vi "UI_Loading_Unit_Test2.vi"() -> ()   [LabVIEW 2014]
panel:
  in  "修改":bool
  in  "加载单元液位过低":bool caption="液位过低"
  in  "加载单元液位过高":bool caption="液位过高"
  in  "加载单元回油过滤器堵塞":bool caption="回油过滤器堵塞"
  in  "加载单元供油过滤器堵塞":bool caption="供油过滤器堵塞"
  out "轴向液压缸加载压力":u16
  out "径向液压缸加载压力":u16
  in  "退出":bool
  in  "系统启动":bool
  out "轴向液压缸加载压力'":dbl(graph) caption="轴向液压缸加载压力"
  out "径向液压缸加载压力'":dbl(graph) caption="径向液压缸加载压力"
  in  "轴向载荷F2":u16
  in  "径向载荷F1":u16
  out "加载单元调试状态":bool
  # "加载单元独立调试"
  # "监测参数"
  # "报警信息"
  # "传\n感\n器"
  # "单\n元\n系\n统"
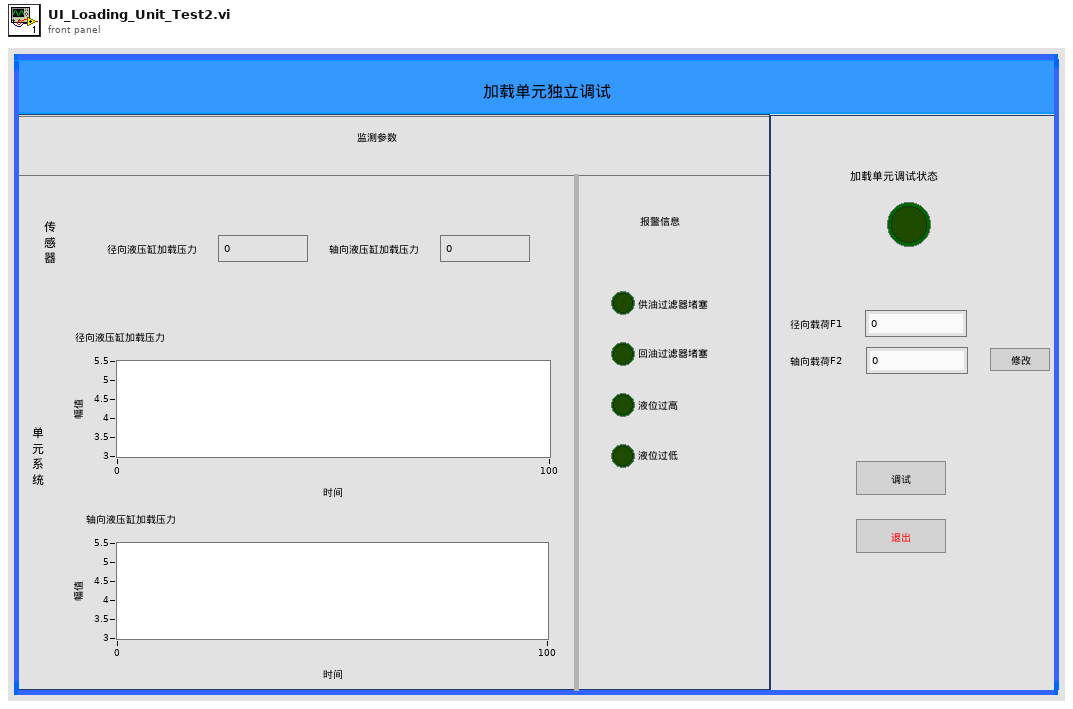
[diagram p1: front panel]
types:
  T1 = cluster{"径向油缸加载压力":u16, "轴向油缸加载压力":u16, "油箱1油液温度":u16, "润滑油温度":u16, "油箱2油液温度":u16, "试验轴承供油压力":u16, "试验轴承供油流量":u16, "陪试轴承供油流量":u16, "陪试轴承供油压力":u16, "陪试轴承供油温度":u16, "液压子系统状态字":cluster{"加载单元":cluster{"供油过滤器堵塞报警":bool, "回油过滤器堵塞报警":bool, "液位过高报警":bool, "液位过低报警":bool}, "试验轴承单元":cluster{"加热装置异常报警":bool, "油箱1液位过高报警":bool, "油箱1液位过低报警":bool, "油箱2液位过高报警":bool, "油箱2液位过低报警":bool, "供油过滤器堵塞报警":bool, "循环回路过滤器堵塞报警":bool, "回油过滤器堵塞报警":bool}, "陪试轴承单元":cluster{"供油过滤器1堵塞报警":bool, "供油过滤器2堵塞报警":bool, "回油过滤器堵塞报警":bool, "油箱液位过高报警":bool, "油箱液位过低报警":bool}}}
  T2 = cluster{"供油过滤器堵塞报警":bool, "回油过滤器堵塞报警":bool, "液位过高报警":bool, "液位过低报警":bool}
  T3 = cluster{"时间":timestamp, "陪试轴承润滑单元出油温度1":sgl[], "陪试轴承润滑单元出油温度2":sgl[], "轴承外圈温度":sgl[], "出油温度":sgl[], "摩擦力1":sgl[], "摩擦力2":sgl[], "径向油缸力":sgl[], "轴向油缸力":sgl[], "转速":sgl[]}
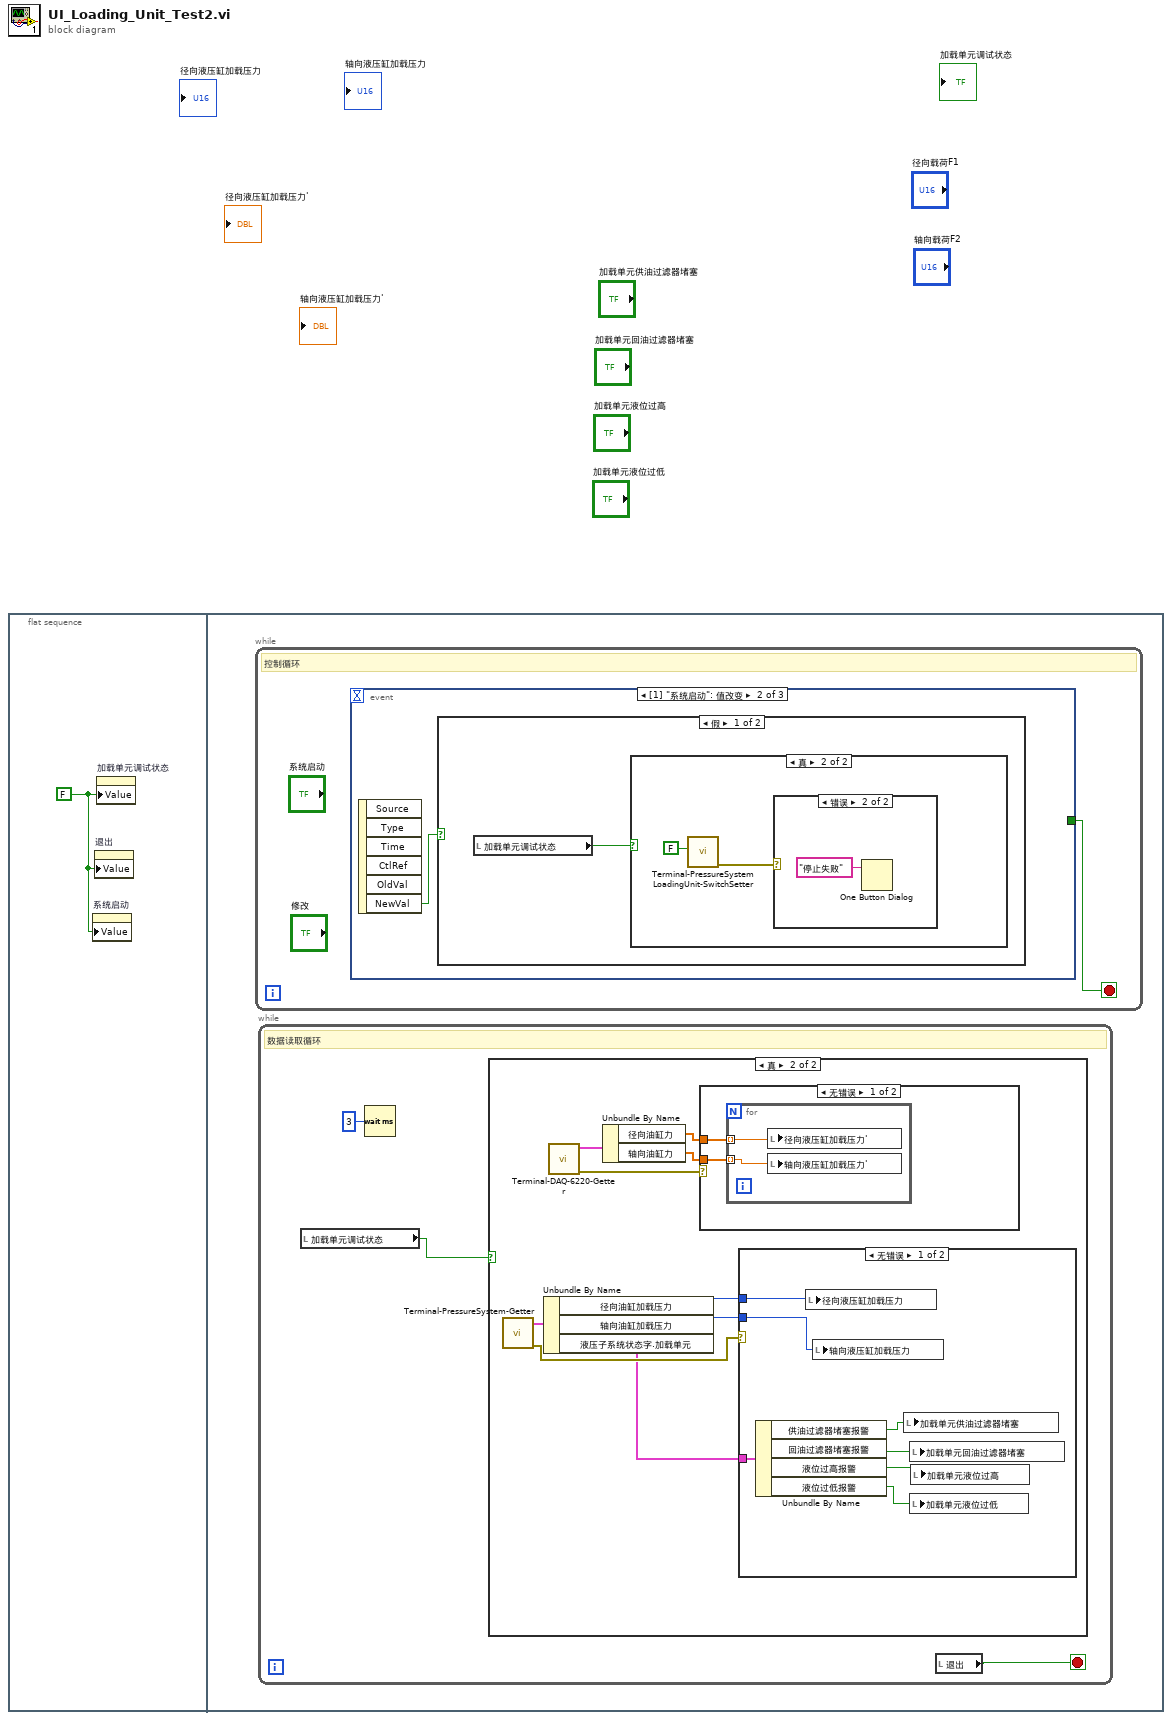
[diagram p0: block diagram]
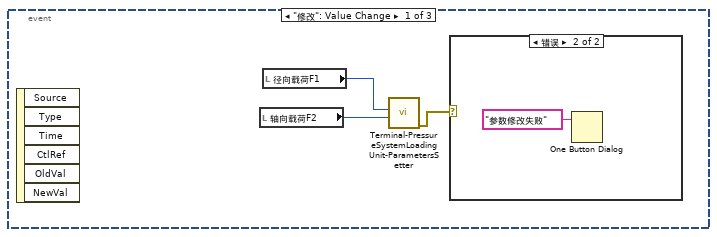
[diagram p5: hidden frame]
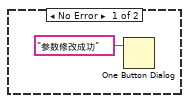
[diagram p6: hidden frame]
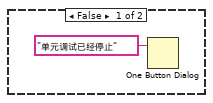
[diagram p7: hidden frame]
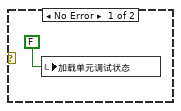
[diagram p8: hidden frame]
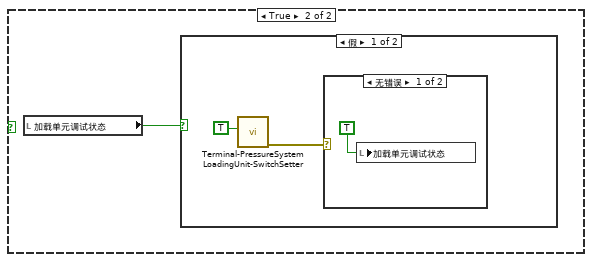
[diagram p9: hidden frame]
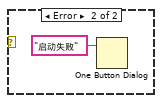
[diagram p10: hidden frame]
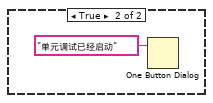
[diagram p11: hidden frame]
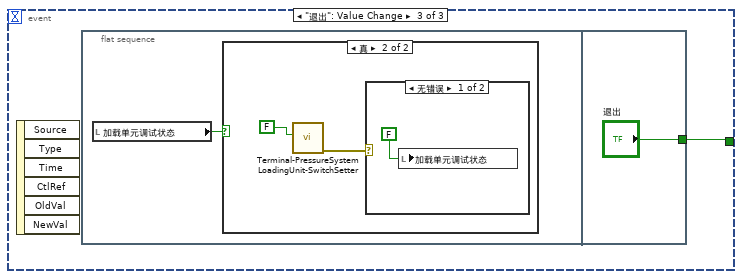
[diagram p12: hidden frame]
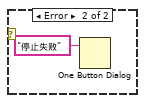
[diagram p14: hidden frame]
diagram:
  n1 = flat-sequence {
    frame #0 {
      w1 = FALSE ("加载单元调试状态")
      n2 = property on="系统启动" class="Bool (严格)"("Value"=w1) -> ()  [unwired: 2 in, 2 out]
      n3 = property on="退出" class="Bool (严格)"("Value"=w1) -> ()  [unwired: 2 in, 2 out]
      n4 = property on="加载单元调试状态" class="Bool (严格)"("Value"=w1) -> ()  [unwired: 2 in, 2 out]
    }
    frame #1 {
      n5 = while {
        stop <- w25 stop-if-true
        # "控制循环"
        n6 = event shown="[1] \"系统启动\": 值改变" {
          selector: _ -> [_ _ _]
          dyn-events: _ -> [_ _ _]
          timeout: _ -> [_ _ _]
          tunnel: [_ _ w44] -> w25
          event "修改": Value Change {
            n7 = event-data() -> ()  [unwired: 1 in, 6 out]
            n8 = local read "轴向载荷F2"() -> (w27:u16)
            n9 = local read "径向载荷F1"() -> (w28:u16)
            n10 = call "Terminal-PressureSystemLoadingUnit-ParametersSetter.vi"("轴向载荷F2"=w27, "径向载荷F1"=w28) -> ("error out"=w26:errorcluster)  [unwired: 9 in]
            n11 = case shown="错误" w26 {
              frame No Error {
                n12 = One Button Dialog(message="参数修改成功" ("消息")) -> ()  [unwired: 1 in, 1 out]
              }
              frame Error {
                n13 = One Button Dialog(message="参数修改失败" ("消息")) -> ()  [unwired: 1 in, 1 out]
              }
            }
          }
          event "系统启动": Value Change {
            n14 = event-data() -> ("NewVal"=w31:bool)  [unwired: 1 in, 5 out]
            n15 = case shown="假" w31 {
              frame False {
                n16 = local read "加载单元调试状态"() -> (w32:bool)
                n17 = case shown="真" w32 {
                  frame False {
                    n18 = One Button Dialog(message="单元调试已经停止" ("消息")) -> ()  [unwired: 1 in, 1 out]
                  }
                  frame True {
                    n19 = call "Terminal-PressureSystemLoadingUnit-SwitchSetter.vi"("启停"=FALSE) -> ("error out"=w34:errorcluster)  [unwired: 10 in]
                    n20 = case shown="错误" w34 {
                      frame No Error {
                        n21 = local write "加载单元调试状态"(FALSE) -> ()
                      }
                      frame Error {
                        n22 = One Button Dialog(message="停止失败" ("消息")) -> ()  [unwired: 1 in, 1 out]
                      }
                    }
                  }
                }
              }
              frame True {
                n23 = local read "加载单元调试状态"() -> (w38:bool)
                n24 = case shown="假" w38 {
                  frame False {
                    n25 = call "Terminal-PressureSystemLoadingUnit-SwitchSetter.vi"("启停"=TRUE) -> ("error out"=w39:errorcluster)  [unwired: 10 in]
                    n26 = case shown="无错误" w39 {
                      frame No Error {
                        n27 = local write "加载单元调试状态"(TRUE) -> ()
                      }
                      frame Error {
                        n28 = One Button Dialog(message="启动失败" ("消息")) -> ()  [unwired: 1 in, 1 out]
                      }
                    }
                  }
                  frame True {
                    n29 = One Button Dialog(message="单元调试已经启动" ("消息")) -> ()  [unwired: 1 in, 1 out]
                  }
                }
              }
            }
          }
          event "退出": Value Change {
            n30 = event-data() -> ()  [unwired: 1 in, 6 out]
            n31 = flat-sequence {
              tunnel: ["退出"] -> w44
              frame #0 {
                n32 = local read "加载单元调试状态"() -> (w45:bool)
                n33 = case shown="真" w45 {
                  frame False {
                  }
                  frame True {
                    n34 = call "Terminal-PressureSystemLoadingUnit-SwitchSetter.vi"("启停"=FALSE) -> ("error out"=w47:errorcluster)  [unwired: 10 in]
                    n35 = case shown="无错误" w47 {
                      frame No Error {
                        n36 = local write "加载单元调试状态"(FALSE) -> ()
                      }
                      frame Error {
                        n37 = One Button Dialog(message="停止失败" ("消息")) -> ()  [unwired: 1 in, 1 out]
                      }
                    }
                  }
                }
              }
              frame #1 {
              }
            }
          }
        }
      }
      n38 = while {
        stop <- w3 stop-if-true
        # "数据读取循环"
        n39 = local read "加载单元调试状态"() -> (w4:bool)
        n40 = Wait (ms)(milliseconds to wait=u32 3 ("等待时间（毫秒）")) -> ()  [unwired: 1 out]
        n41 = case shown="真" w4 {
          frame False {
          }
          frame True {
            n42 = call "Terminal-PressureSystem-Getter.vi"() -> ("error out"=w9:errorcluster, "设备信息"=w8:T1)  [unwired: 10 in]
            n43 = Unbundle By Name(w8) -> ("径向油缸加载压力"=w7:u16, "轴向油缸加载压力"=w6:u16, "液压子系统状态字.加载单元"=w5:T2)
            n44 = call "Terminal-DAQ-6220-Getter.vi"() -> ("error out"=w13:errorcluster, "6220"=w12:T3)  [unwired: 10 in]
            n45 = Unbundle By Name(w12) -> ("径向油缸力"=w11:sgl[], "轴向油缸力"=w10:sgl[])
            n46 = case shown="无错误" w13 {
              tunnel: w11 -> [w22 _]
              tunnel: w10 -> [w21 _]
              frame No Error {
                n47 = for {
                  tunnel: w22 -> [w24] mode=indexing
                  tunnel: w21 -> [w23] mode=indexing
                  n48 = local write "径向液压缸加载压力'"(w24) -> ()
                  n49 = local write "轴向液压缸加载压力'"(w23) -> ()
                }
              }
              frame Error {
              }
            }
            n50 = case shown="无错误" w9 {
              tunnel: w7 -> [w20 _]
              tunnel: w6 -> [w19 _]
              tunnel: w5 -> [w18 _]
              frame No Error {
                n51 = Unbundle By Name(w18) -> ("供油过滤器堵塞报警"=w17:bool, "回油过滤器堵塞报警"=w16:bool, "液位过高报警"=w15:bool, "液位过低报警"=w14:bool)
                n52 = local write "径向液压缸加载压力"(w20) -> ()
                n53 = local write "轴向液压缸加载压力"(w19) -> ()
                n54 = local write "加载单元供油过滤器堵塞"(w17) -> ()
                n55 = local write "加载单元回油过滤器堵塞"(w16) -> ()
                n56 = local write "加载单元液位过低"(w14) -> ()
                n57 = local write "加载单元液位过高"(w15) -> ()
              }
              frame Error {
              }
            }
          }
        }
        n58 = local read "退出"() -> (w3:bool)
      }
    }
  }
